vi "OE1022D_Configure Sample.vi"(7 "OE1022D_Configure Sample":T1={"Trigger Mode"=0, "Sample Mode"=0, "Sample Time(ms)"=100, "Length"=50, "Channel"=1, "Sample State"=0, "Buffer 1"=0, "Buffer 2"=1, "Buffer 3"=2, "Buffer 4"=3} {"Buffer 4" items=["R", "X", "Y", "Theta", "Rh1", "Xh1", "Yh1", "Theta h1", "Rh2", "Xh2", "Yh2", "Theta h2", "Noise", "A1", "A2", "A3", "A4", "E1", "E2", "E3", "E4", "Freq"]; "Buffer 3" items=["R", "X", "Y", "Theta", "Rh1", "Xh1", "Yh1", "Theta h1", "Rh2", "Xh2", "Yh2", "Theta h2", "Noise", "A1", "A2", "A3", "A4", "E1", "E2", "E3", "E4", "Freq"]; "Buffer 2" items=["R", "X", "Y", "Theta", "Rh1", "Xh1", "Yh1", "Theta h1", "Rh2", "Xh2", "Yh2", "Theta h2", "Noise", "A1", "A2", "A3", "A4", "E1", "E2", "E3", "E4", "Freq"]; "Buffer 1" items=["R", "X", "Y", "Theta", "Rh1", "Xh1", "Yh1", "Theta h1", "Rh2", "Xh2", "Yh2", "Theta h2", "Noise", "A1", "A2", "A3", "A4", "E1", "E2", "E3", "E4", "Freq"]; "Sample State" items=["Start", "Pause", "Stop and Clear"]; "Channel" items=["A"=1, "B"=2]; "Length" min=1 max=16384; "Sample Time(ms)" min=1 max=100000; "Sample Mode" items=["Single", "Loop"]; "Trigger Mode" items=["Int", "Ext"]}, 8 "Error in (no error)":errorcluster caption="error out（no error）", 9 "Remote Mode":u16(ring) items=["USB", "RS232", "GPIB"], 11 "VISA resource name":refnum<visa-resource-name>) -> (0 "Error out":errorcluster caption="error out", 1 "Output String":string, 3 "VISA resource  out":refnum<visa-resource-name>)   [LabVIEW 2011]
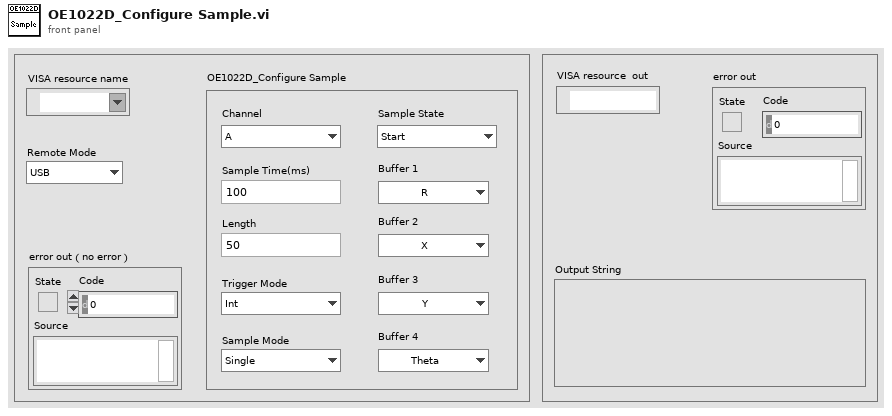
[diagram p1: front panel]
types:
  T1 = cluster{"Trigger Mode":u16, "Sample Mode":u16, "Sample Time(ms)":u32, "Length":u16, "Channel":u16, "Sample State":u16, "Buffer 1":u16, "Buffer 2":u16, "Buffer 3":u16, "Buffer 4":u16}
  T2 = enum16{"ISRC", "IGND", "ICPL", "ILIN", "PHAS", "FMOD", "RSLP", "FREQ", "SWPT", "SLLM", "SULM", "SSLL", "SSLG", "STLM", "SWRM", "IRNG", "SENS", "RMOD", "OFLT", "OFSL", "SYNC", "DMOD", "HARM", "DARB", "SWVT", "SLVL", "SVLL", "SVUL", "SVSL", "SVSG", "SVTM", "SVRM", "RALL", "SNAP", "OUTP", "OAUX", "COUT", "CAUX", "COFP", "CEXP", "FPOP", "OEXP", "*IDN", "*RST", "OVLD", "INOV", "GNOV", "*PLL", "SSET", "RSET", "AGAN", "APHS", "ARSV", "ASCL", "EQCD", "EQCS", "SPED", "SRAT", "SLEN", "SSLE", "STRG", "SPRM", "STRD", "PAUS", "REST", "SPTS", "TRCA", "TEMP", "RSTU", "IHNZ", "DEQU", "SADD", "ARNG", "CSPE", "ISRCD", "IGNDD", "ICPLD", "ILIND", "PHASD", "FMODD", "RSLPD", "FREQD", "SWPTD", "SLLMD", "SULMD", "SSLLD", "SSLGD", "STLMD", "SWRMD", "SENSD", "RMODD", "OFLTD", "OFSLD", "SYNCD", "HARMD", "EQCDD", "EQCSD", "SNAPD", "OUTPD", "SWVTD", "SLVLD", "SVLLD", "SVULD", "SVSLD", "SVSGD", "SVTMD", "SVRMD", "SVDCD", "ARSVD", "AGAND", "APHSD", "ASCLD", "FPOPD", "CAUXD", "OEXPD", "SPEDD", "SRATD", "SLEND", "SSLED", "STRGD", "SPRMD", "STRDD", "PAUSD", "RESTD", "SPTSD", "TRCAD", "*IDND", "*RSTD", "INOVD", "GNOVD", "*PLLD", "SSETD", "RSETD"}
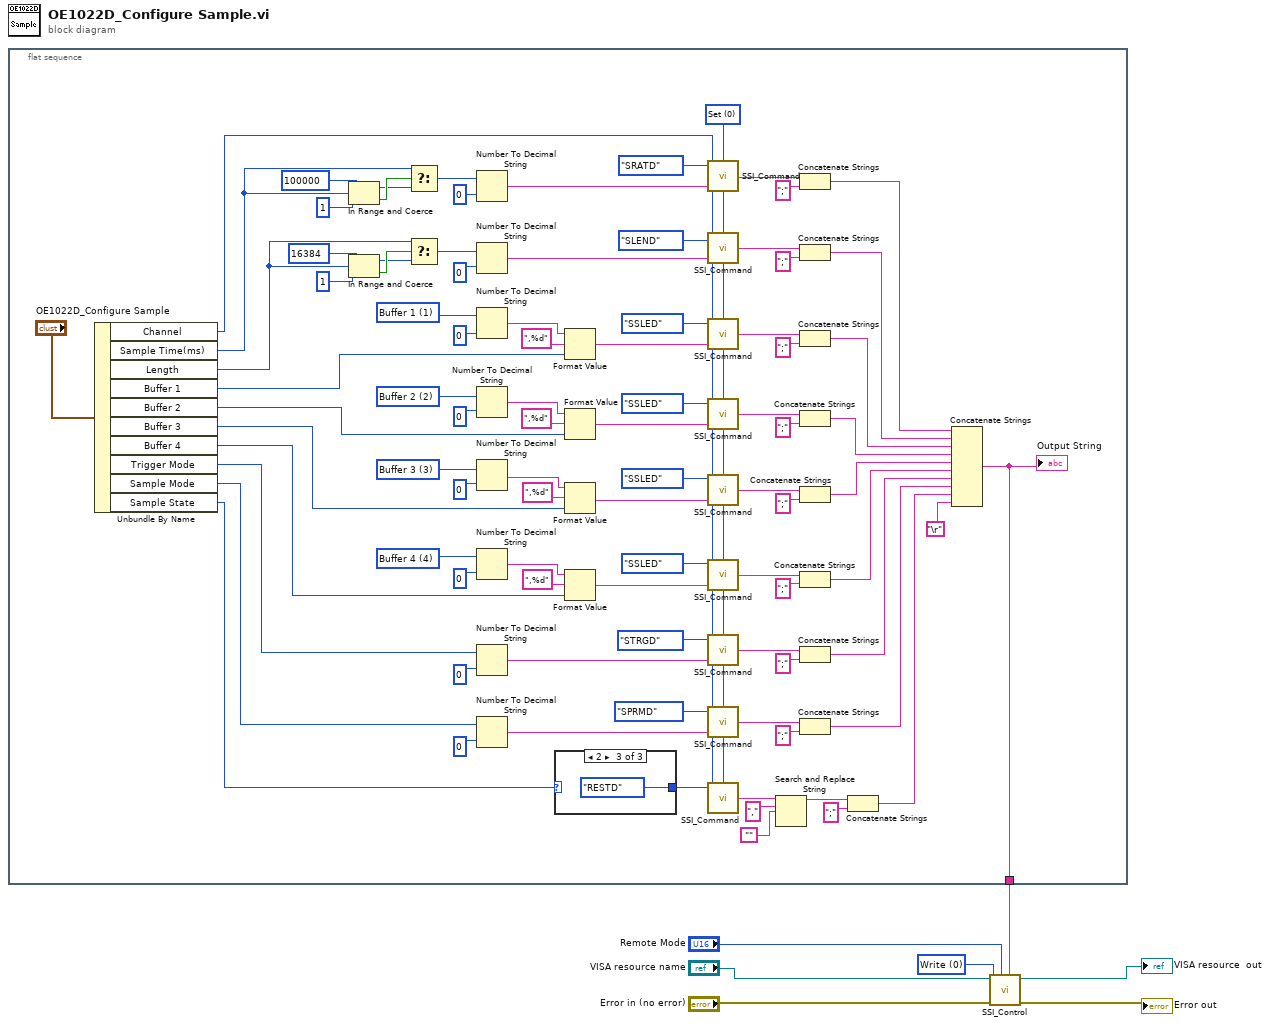
[diagram p0: block diagram]
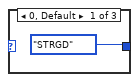
[diagram p2: hidden frame]
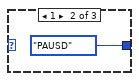
[diagram p3: hidden frame]
diagram:
  w6 = u16 0 items=["Write", "Read"] ("Control")
  n1 = flat-sequence {
    tunnel: [w92] -> w1
    frame #0 {
      w49 = u16 4 items=["Buffer 1"=1, "Buffer 2"=2, "Buffer 3"=3, "Buffer 4"=4]
      w60 = u16 3 items=["Buffer 1"=1, "Buffer 2"=2, "Buffer 3"=3, "Buffer 4"=4]
      w65 = u16 2 items=["Buffer 1"=1, "Buffer 2"=2, "Buffer 3"=3, "Buffer 4"=4]
      w15 = u16 0 items=["Set", "Query"] ("Opera")
      w70 = u16 1 items=["Buffer 1"=1, "Buffer 2"=2, "Buffer 3"=3, "Buffer 4"=4]
      n2 = Unbundle By Name("OE1022D_Configure Sample") -> ("Channel"=w14:u16, "Sample Time(ms)"=w57:u32, "Length"=w55:u16, "Buffer 1"=w68:u16, "Buffer 2"=w64:u16, "Buffer 3"=w59:u16, "Buffer 4"=w50:u16, "Trigger Mode"=w53:u16, "Sample Mode"=w54:u16, "Sample State"=w13:u16)
      n3 = In Range and Coerce(upper limit=u32 100000 ("上限"), x=w57, lower limit=u32 1 ("下限")) -> (coerced(x)=w96:u32, In Range?=w97:bool)
      n4 = In Range and Coerce(upper limit=u16 16384 ("上限"), x=w55, lower limit=u16 1 ("下限")) -> (coerced(x)=w89:u16, In Range?=w90:bool)
      n5 = Select(t=w57, s=w97, f=w96) -> (s? t:f=w56:u32)
      n6 = Select(t=w55, s=w90, f=w89) -> (s? t:f=w58:u16)
      n7 = Number To Decimal String(number=w56, width (-)=i16 0 ("精度(6)")) -> (decimal integer string=w74:string)
      n8 = Number To Decimal String(number=w58, width (-)=i16 0 ("宽度(-)")) -> (decimal integer string=w73:string)
      n9 = Number To Decimal String(number=w70, width (-)=i16 0 ("宽度(-)")) -> (decimal integer string=w69:string)
      n10 = Number To Decimal String(number=w65, width (-)=i16 0 ("宽度(-)")) -> (decimal integer string=w66:string)
      n11 = Number To Decimal String(number=w60, width (-)=i16 0 ("宽度(-)")) -> (decimal integer string=w61:string)
      n12 = Number To Decimal String(number=w49, width (-)=i16 0 ("宽度(-)")) -> (decimal integer string=w48:string)
      n13 = Number To Decimal String(number=w53, width (-)=i16 0 ("宽度(-)")) -> (decimal integer string=w43:string)
      n14 = Number To Decimal String(number=w54, width (-)=i16 0 ("宽度(-)")) -> (decimal integer string=w44:string)
      n15 = case shown="2" w13 {
        tunnel: [T2."STRGD" ("Command Type") T2."PAUSD" ("Command Type") T2."RESTD" ("Command Type")] -> w12
        frame 0, Default {
        }
        frame 1 {
        }
        frame 2 {
        }
      }
      n16 = Format Value(string ("")=w69, format string=",%d" ("格式字符串"), value (0)=w68) -> (output string=w71:string)
      n17 = Format Value(string ("")=w66, format string=",%d" ("格式字符串"), value (0)=w64) -> (output string=w47:string)
      n18 = Format Value(string ("")=w61, format string=",%d" ("格式字符串"), value (0)=w59) -> (output string=w46:string)
      n19 = Format Value(string ("")=w48, format string=",%d" ("格式字符串"), value (0)=w50) -> (output string=w45:string)
      n20 = call "SSI_Command.vi"("Opera"=w15, "Paramter"=w74, "channel"=w14, "Command Type"=T2."SRATD") -> ("Output string"=w42:string)
      n21 = call "SSI_Command.vi"("Opera"=w15, "Paramter"=w73, "channel"=w14, "Command Type"=T2."SLEND") -> ("Output string"=w37:string)
      n22 = call "SSI_Command.vi"("Opera"=w15, "Paramter"=w71, "channel"=w14, "Command Type"=T2."SSLED") -> ("Output string"=w38:string)
      n23 = call "SSI_Command.vi"("Opera"=w15, "Paramter"=w47, "channel"=w14, "Command Type"=T2."SSLED") -> ("Output string"=w36:string)
      n24 = call "SSI_Command.vi"("Opera"=w15, "Paramter"=w46, "channel"=w14, "Command Type"=T2."SSLED") -> ("Output string"=w34:string)
      n25 = call "SSI_Command.vi"("Opera"=w15, "Paramter"=w45, "channel"=w14, "Command Type"=T2."SSLED") -> ("Output string"=w32:string)
      n26 = call "SSI_Command.vi"("Opera"=w15, "Paramter"=w43, "channel"=w14, "Command Type"=T2."STRGD") -> ("Output string"=w30:string)
      n27 = call "SSI_Command.vi"("Opera"=w15, "Paramter"=w44, "channel"=w14, "Command Type"=T2."SPRMD") -> ("Output string"=w28:string)
      n28 = call "SSI_Command.vi"("Opera"=w15, "channel"=w14, "Command Type"=w12) -> ("Output string"=w18:string)  [unwired: 1 in]
      n29 = Search and Replace String(input string=w18, search string="," ("搜索字符串"), replace string="") -> (result string=w9:string)  [unwired: 5 in, 3 out]
      n30 = Concatenate Strings(w42, ";" ("替换字符串(\"\")")) -> (w26:string)
      n31 = Concatenate Strings(w37, ";" ("替换字符串(\"\")")) -> (w25:string)
      n32 = Concatenate Strings(w38, ";" ("替换字符串(\"\")")) -> (w24:string)
      n33 = Concatenate Strings(w36, ";" ("替换字符串(\"\")")) -> (w23:string)
      n34 = Concatenate Strings(w34, ";" ("替换字符串(\"\")")) -> (w22:string)
      n35 = Concatenate Strings(w32, ";" ("替换字符串(\"\")")) -> (w21:string)
      n36 = Concatenate Strings(w30, ";" ("替换字符串(\"\")")) -> (w20:string)
      n37 = Concatenate Strings(w28, ";" ("替换字符串(\"\")")) -> (w19:string)
      n38 = Concatenate Strings(w9, ";" ("替换字符串(\"\")")) -> (w8:string)
      n39 = Concatenate Strings(w26, w25, w24, w23, w22, w21, w20, w19, w8, "\r") -> (w92:string)
      "Output String" <- w92
    }
  }
  n40 = call "SSI_Control.vi"("Write Buffer"=w1, "Remote Mode"="Remote Mode", "Error in (no error)"="Error in (no error)", "Control"=w6, "VISA resource name"="VISA resource name") -> ("Error out"=→"Error out":errorcluster, "VISA resource  out"=→"VISA resource  out":refnum<visa-resource-name>)  [unwired: 3 in, 2 out]
